vi "RFH-convert-water_calib_file.vi"() -> ()   [LabVIEW 2020, in "RFH-Reflection_File_Handler.lvlib"]
uses:
  RFH-Reflection_File_Handler.lvlib
  RFH-common_data_format.ctl
panel:
  out "error out":errorcluster
  in  "Water temp C":dbl=25.0
  in  "Save Name":string
  in  "Save Path":path
  in  "LibreVNA samplerate file":path
  in  "Water filepath":path
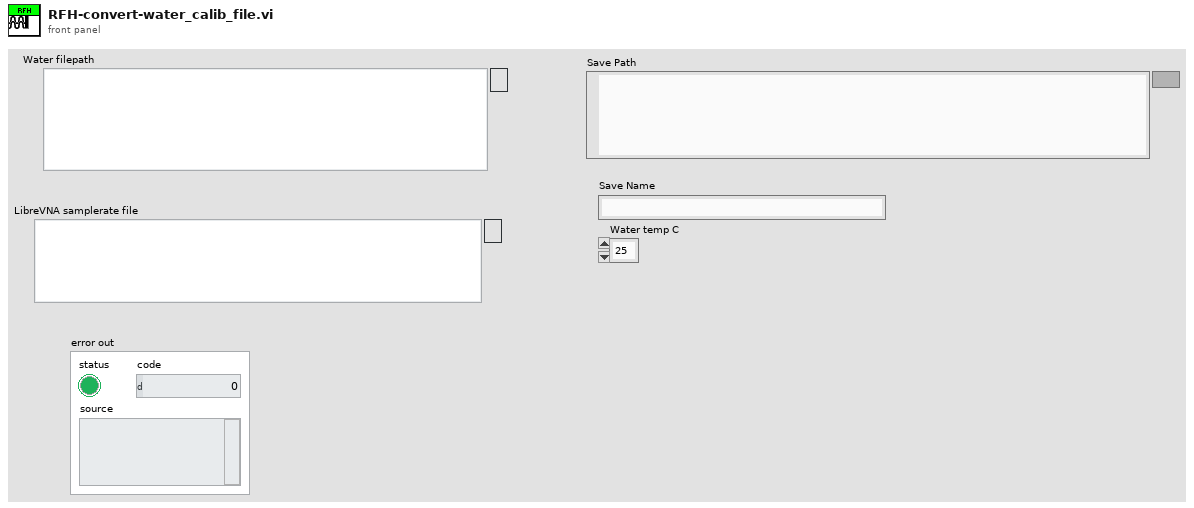
[diagram p1: front panel]
types:
  T1 = typedef "RFH-Reflection_File_Handler.lvlib/RFH-common_data_format.ctl" = cluster{"Frequency":dbl[], "Reflection'":dbl[], "Reflection''":dbl[], "Permativity'":dbl[], "Permativity''":dbl[]}
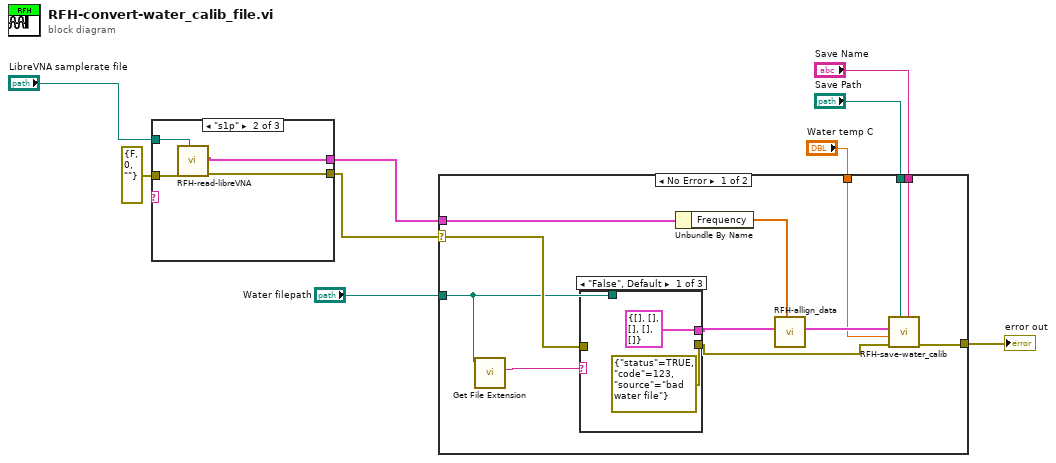
[diagram p0: block diagram]
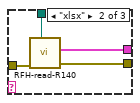
[diagram p2: hidden frame]
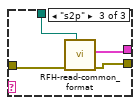
[diagram p3: hidden frame]
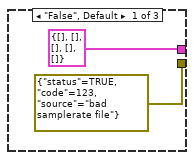
[diagram p5: hidden frame]
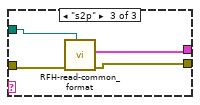
[diagram p6: hidden frame]
diagram:
  n1 = case shown="\"s1p\"" {
    selector: _ -> [_ _ _]
    tunnel: [T1 {"Frequency"=[], "Reflection'"=[], "Reflection''"=[], "Permativity'"=[], "Permativity''"=[]} ("Common Format") w12 w18] -> w1
    tunnel: [errorcluster {"status"=TRUE, "code"=123, "source"="bad samplerate file"} ("error out") w13 w17] -> w2
    tunnel: errorcluster {"status"=FALSE, "code"=0, "source"=""} ("error out") -> [_ w14 w19]
    tunnel: "LibreVNA samplerate file" -> [_ w15 w16]
    frame "False", Default {
    }
    frame "s1p" {
      n2 = call "RFH-read-libreVNA.vi"("file path (dialog if empty)"=w15, "error in"=w14) -> ("error out"=w13:errorcluster, "Common Format"=w12:T1)  [unwired: 8 in]
    }
    frame "s2p" {
      n3 = call "RFH-read-common_format.vi"("file path (dialog if empty)"=w16, "error in"=w19) -> ("error out"=w17:errorcluster, "Common Format"=w18:T1)  [unwired: 8 in]
    }
  }
  n4 = case shown="No Error" w2 {
    selector: w2 -> [w22 w42]
    tunnel: w1 -> [w30 _]
    tunnel: "Save Path" -> [w27 _]
    tunnel: "Save Name" -> [w26 _]
    tunnel: "Water temp C" -> [w25 _]
    tunnel: [w23 w42] -> w6
    tunnel: "Water filepath" -> [w21 _]
    frame No Error {
      n5 = call <vilib>:"Get File Extension.vi"("file"=w21) -> ("lowercase file extension"=w20:string)  [unwired: 6 in, 4 out]
      n6 = case shown="\"False\", Default" w20 {
        tunnel: [T1 {"Frequency"=[], "Reflection'"=[], "Reflection''"=[], "Permativity'"=[], "Permativity''"=[]} ("Common Format") w37 w39] -> w31
        tunnel: w21 -> [_ w36 w40]
        tunnel: [errorcluster {"status"=TRUE, "code"=123, "source"="bad water file"} ("error out") w35 w38] -> w24
        tunnel: w22 -> [_ w34 w41]
        frame "False", Default {
        }
        frame "xlsx" {
          n7 = call "RFH-read-R140.vi"("file path (dialog if empty)"=w36, "error in (no error)"=w34) -> ("error out"=w35:errorcluster, "Common Format"=w37:T1)  [unwired: 7 in, 1 out]
        }
        frame "s2p" {
          n8 = call "RFH-read-common_format.vi"("file path (dialog if empty)"=w40, "error in"=w41) -> ("error out"=w38:errorcluster, "Common Format"=w39:T1)  [unwired: 8 in]
        }
      }
      n9 = Unbundle By Name(w30) -> ("Frequency"=w29:dbl[])
      n10 = call "RFH-allign_data.vi"("Xi"=w29, "Common Format"=w31) -> ("Common Format alligned"=w28:T1)  [unwired: 9 in]
      n11 = call "RFH-save-water_calib.vi"("Save Name"=w26, "Save Path"=w27, "error in (no error)"=w24, "Water temp"=w25, "Common Format"=w28) -> ("error out"=w23:errorcluster)  [unwired: 6 in]
    }
    frame Error {
    }
  }
  "error out" <- w6
